vi "read config file.vi"(8 "error in (no error)":errorcluster, 11 "Header content in":refnum<class "Header content.lvclass">) -> (0 "error out":errorcluster, 2 "remote IPs":string[](array[string]), 3 "Header content out":refnum<class "Header content.lvclass">)   [LabVIEW 2018, in "Header content.lvclass"]
uses:
  Header content.lvclass
  <vilib>/Utility/config.llb/Read Key (String).vi
  <vilib>/Utility/config.llb/NI_LVConfig.lvlib
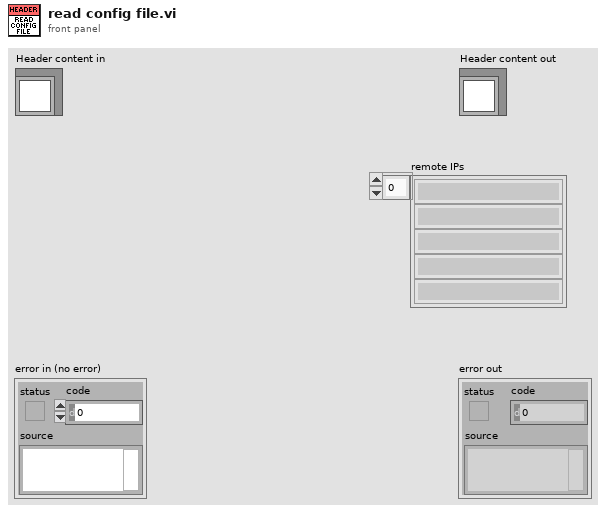
[diagram p1: front panel]
types:
  T1 = typedef "NI_LVConfig.lvlib/Config Data RefNum.ctl" = refnum<k1>
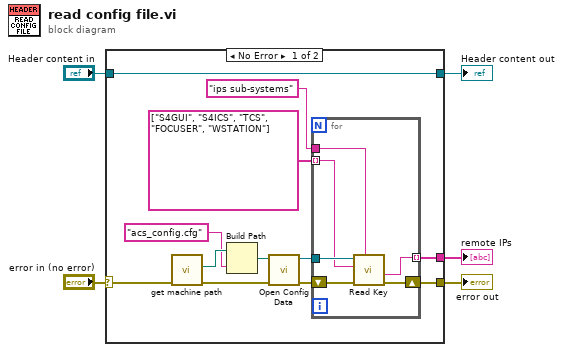
[diagram p0: block diagram]
diagram:
  n1 = case shown="No Error" "error in (no error)" {
    selector: "error in (no error)" -> [w10 w25]
    tunnel: [w15 w25] -> w4
    tunnel: [w17 w24] -> w2
    tunnel: "Header content in" -> [w17 w24]
    tunnel: [w11 _] -> w1
    frame No Error {
      n2 = call "get machine path.vi"("error in (no error) 2"=w10) -> ("error in (no error)"=w9:errorcluster, "machine path"=w8:path)  [unwired: 9 in]
      n3 = Build Path(base path=w8, name or relative path="acs_config.cfg") -> (appended path=w7:path)
      n4 = call <vilib>:"Open Config Data.vi"("error in (no error)"=w9, "configuration file path"=w7) -> ("error out"=w16:errorcluster, "refnum"=w14:T1)  [unwired: 7 in, 1 out]
      n5 = for {
        tunnel: w14 -> [w21]
        tunnel: "ips sub-systems" ("section") -> [w20]
        shift-right: [w22] -> w15
        shift-left: w16 -> [w23]
        tunnel: string[] ["S4GUI", "S4ICS", "TCS", "FOCUSER", "WSTATION"] -> [w19] mode=indexing
        tunnel: [w18] -> w11 mode=indexing
        n6 = call-poly <vilib>:"Read Key.vi"("section"=w20, "error in (no error)"=w23, "key"=w19, "refnum"=w21) -> ("error out"=w22:errorcluster, "value"=w18:string)  [unwired: 4 in, 2 out]
      }
    }
    frame Error {
    }
  }
  "error out" <- w4
  "Header content out" <- w2
  "remote IPs" <- w1
